vi "ForceAngleTo_0_180.vi"(8 "error in (no error)":errorcluster, 11 "Angle in":refnum<class "Angle.lvclass">) -> (0 "error out":errorcluster, 2 "Angle out":dbl)   [LabVIEW 2013, in "Angle.lvclass"]
uses:
  Angle.lvclass
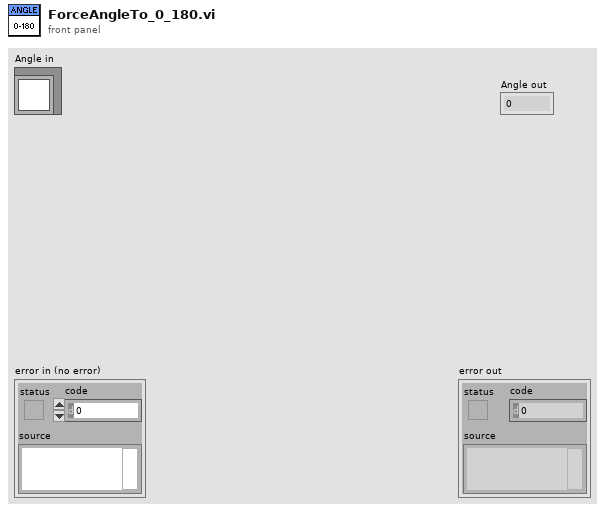
[diagram p1: front panel]
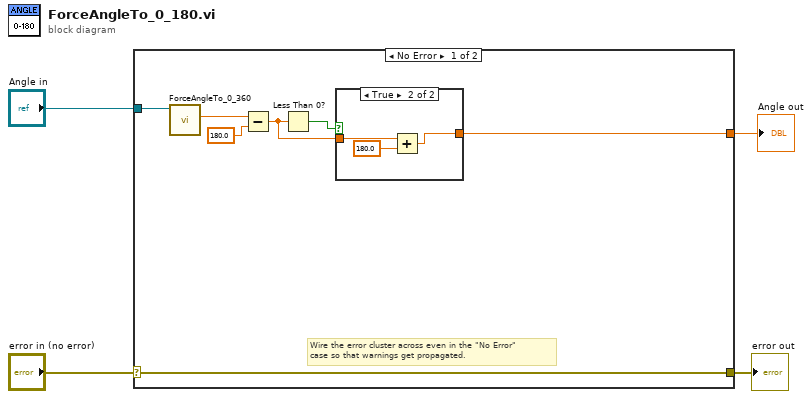
[diagram p0: block diagram]
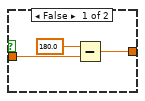
[diagram p2: hidden frame]
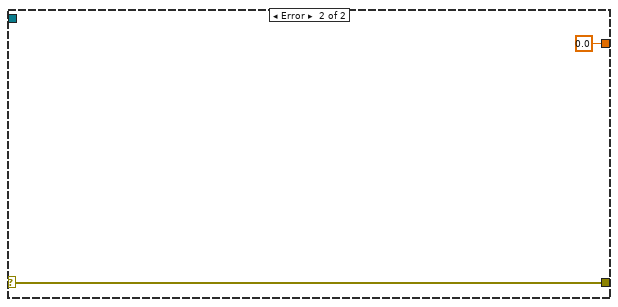
[diagram p3: hidden frame]
diagram:
  n1 = case shown="No Error" "error in (no error)" {
    selector: "error in (no error)" -> [w11 w19]
    tunnel: [w11 w19] -> w3
    tunnel: "Angle in" -> [w10 _]
    tunnel: [w5 0.0] -> w1
    frame No Error {
      # "Wire the error cluster across even in the \"No Error\"\ncase so that warnings get propagated."
      n2 = call "ForceAngleTo_0_360.vi"("Angle in"=w10) -> ("Relative Angle"=w9:dbl)  [unwired: 9 in, 1 out]
      n3 = Subtract(x=w9, y=180.0) -> (x-y=w6:dbl)
      n4 = Less Than 0?(x=w6) -> (x < 0?=w7:bool)
      n5 = case shown="True" w7 {
        tunnel: w6 -> [w13 w17]
        tunnel: [w12 w15] -> w5
        frame False {
          n6 = Subtract(x=180.0, y=w13) -> (x-y=w12:dbl)
        }
        frame True {
          n7 = Add(x=w17, y=180.0) -> (x+y=w15:dbl)
        }
      }
    }
    frame Error {
    }
  }
  "error out" <- w3
  "Angle out" <- w1
